vi "extract_trace.vi"(8 "error in (no error)":errorcluster, 9 "sub-pixels per cell":i32=1, 10 "trace index":i32, 11 "ImageCollection in":refnum<class "ImageCollection.lvclass">) -> (0 "error out":errorcluster, 2 "traces":sgl[](graph))   [LabVIEW 2010]
uses:
  common/classes/ImageCollection/ImageCollection/ImageCollection.lvclass
  common/classes/Image/Image/Image.lvclass
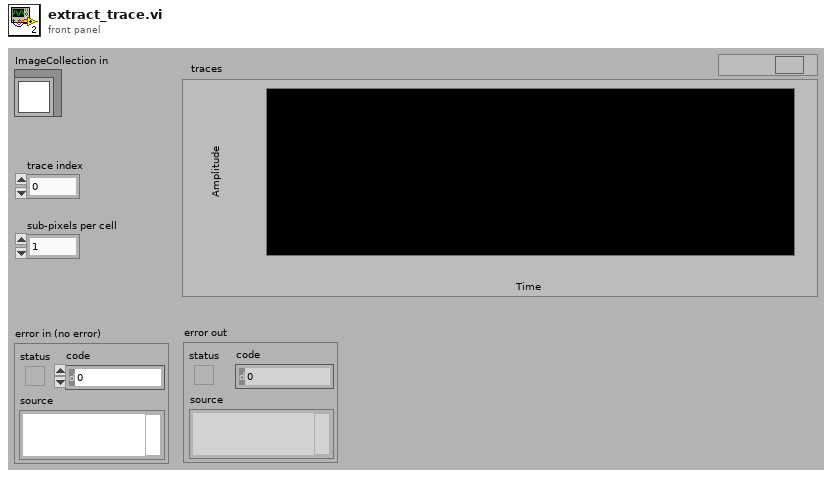
[diagram p1: front panel]
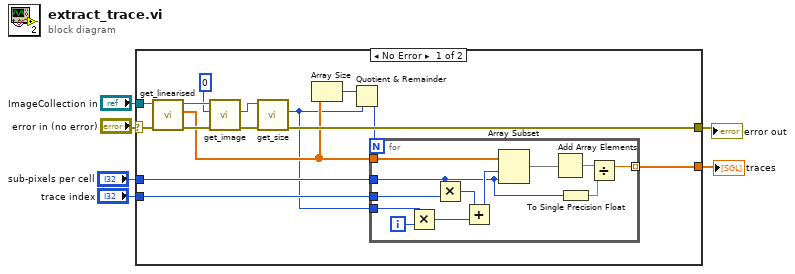
[diagram p0: block diagram]
diagram:
  n1 = case shown="No Error" "error in (no error)" {
    selector: "error in (no error)" -> [w21 w34]
    tunnel: "ImageCollection in" -> [w20 _]
    tunnel: "trace index" -> [w19 _]
    tunnel: [w13 w34] -> w3
    tunnel: "sub-pixels per cell" -> [w10 _]
    tunnel: [w8 _] -> w1
    frame No Error {
      n2 = call "get_linearised.vi"("error in (no error)"=w21, "ImageCollection in"=w20) -> ("error out"=w16:errorcluster, "pixels"=w12:sgl[], "ImageCollection out"=w18:refnum<class "ImageCollection.lvclass">)  [unwired: 7 in]
      n3 = call-dynamic "get_image.vi"("error in (no error)"=w16, "index"=0, "ImageCollection in"=w18) -> ("error out"=w14:errorcluster, "Image.lvclass"=w15:refnum<class "Image.lvclass">)  [unwired: 6 in, 1 out]
      n4 = call-dynamic "get_size.vi"("error in (no error)"=w14, "Image in"=w15) -> ("error out"=w13:errorcluster, "x resolution"=w7:i32)  [unwired: 2 in, 6 out]
      n5 = Array Size(array=w12) -> (size(s)=w11:i32)
      n6 = Quotient & Remainder(x=w11, y=w7) -> (floor(x/y)=w9:i32)  [unwired: 1 out]
      n7 = for {
        N: w9 -> [_]
        tunnel: w12 -> [w31]
        tunnel: w19 -> [w25]
        tunnel: w7 -> [w32]
        tunnel: w10 -> [w24]
        tunnel: [w26] -> w8 mode=indexing
        i -> [w33]
        n8 = Multiply(x=w32, y=w33) -> (x*y=w22:i32)
        n9 = Multiply(x=w24, y=w25) -> (x*y=w23:i32)
        n10 = Add(x=w23, y=w22) -> (x+y=w30:i32)
        n11 = Array Subset(array=w31, index=w30, length=w24) -> (w29:sgl[])
        n12 = Add Array Elements(numeric array=w29) -> (sum=w28:sgl)
        n13 = To Single Precision Float(number=w24) -> (single precision float=w27:sgl)
        n14 = Divide(x=w28, y=w27) -> (x/y=w26:sgl)
      }
    }
    frame Error {
    }
  }
  "error out" <- w3
  "traces" <- w1
